vi "WriteTextFile.vi"(5 "overwrite? (F)":bool, 7 "InitialCali.":dbl[](array[numeric])=[-1.0, -1.0, -1.0], 8 "error in (no error)":errorcluster, 10 "Signal Segment":T1={"SampleRate"=-1.0, "TrigDelay"=0.0, "SpecLength"=0.0, "DAQ_Range"=0.0, "Average#"=0, "Position"=[], "Spectrum"=[], "Calibr."=[], "Pressure"=-1.0, "Desp_LaserEnergy"=-1.0, "PI_LaserEnergy"=-1.0, "Voltages Table"=[], "ProcMode"=enum."None", "Threshold"=-1.0, "Comment"="", "TickCount"=0.0, "Time Stamp"=timestamp(0 s since 1904-01-01)} {"TickCount" format="%#.2f"}, 11 "Filename":path) -> (0 "error out":errorcluster)   [LabVIEW 2013]
uses:
  Signal_Segment.ctl
  ControlDef/ProcessingMode.ctl
  <vilib>/Utility/error.llb/DialogType.ctl
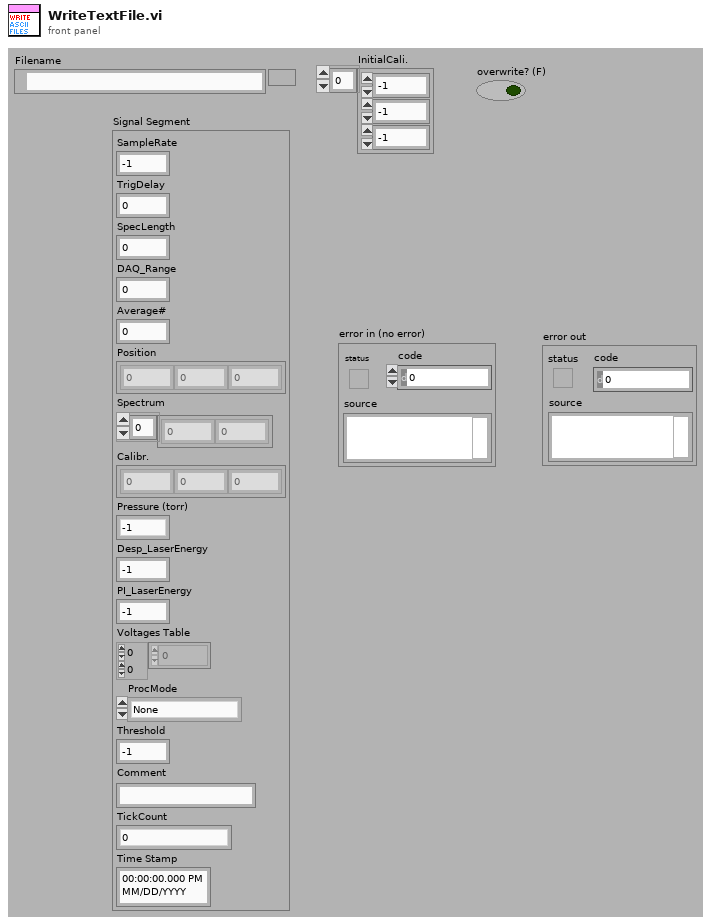
[diagram p1: front panel]
types:
  T1 = typedef "Signal_Segment.ctl" = cluster{"SampleRate":dbl, "TrigDelay":dbl, "SpecLength":dbl, "DAQ_Range":dbl, "Average#":i32, "Position":dbl[], "Spectrum":sgl[], "Calibr.":dbl[], "Pressure":dbl, "Desp_LaserEnergy":dbl, "PI_LaserEnergy":dbl, "Voltages Table":sgl[][], "ProcMode":T2, "Threshold":dbl, "Comment":string, "TickCount":dbl, "Time Stamp":timestamp}
  T2 = typedef "ProcessingMode.ctl" = enum16{"None", "Drop by Threshold", "TDC Simulate", "SetFilter"}
  T3 = enum16{"open", "replace", "create", "open or create", "replace or create", "replace or create with confirmation"}
  T4 = typedef "DialogType.ctl" = u16
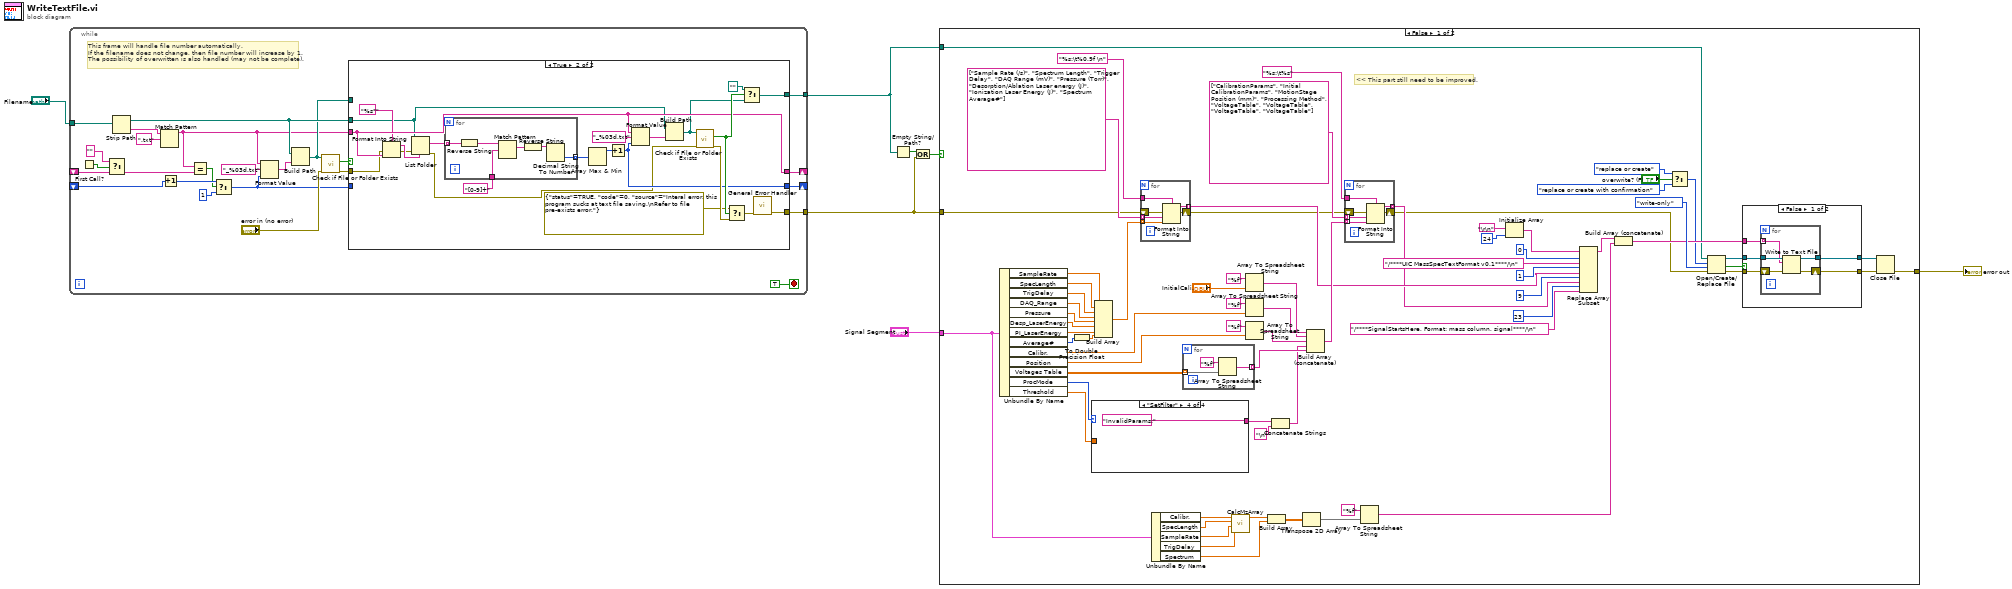
[diagram p0: block diagram]
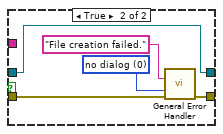
[diagram p3: hidden frame]
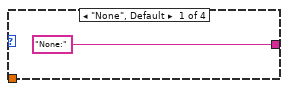
[diagram p4: hidden frame]
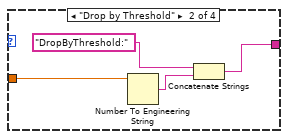
[diagram p5: hidden frame]
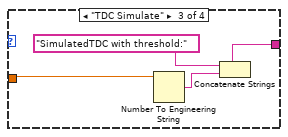
[diagram p6: hidden frame]
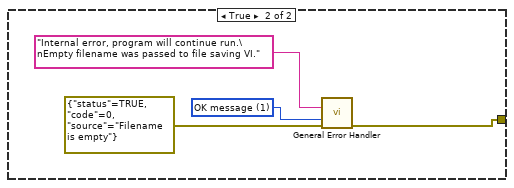
[diagram p7: hidden frame]
diagram:
  n1 = while {
    tunnel: "Filename" -> [w30]
    shift-right: [w23] -> _
    shift-left: _ -> [w10]
    shift-right: [w13] -> _
    shift-left: _ -> [w28]
    tunnel: [w21] -> w3
    tunnel: [w20] -> w1
    stop <- TRUE stop-if-true
    # "This frame will handle file number automatically.\nIf the filename does not change, then file number will increase by 1.\nThe possibility of overwritten is also handled (may not be complete)."
    n2 = First Call?() -> (First Call?: T/F=w9:bool)
    n3 = Select(t="", s=w9, f=w10) -> (s? t:f=w11:string)
    n4 = Strip Path(path=w30) -> (stripped path=w22:path, name=w32:string)
    n5 = Match Pattern(string=w32, regular expression=".txt") -> (before substring=w15:string)  [unwired: 1 in, 3 out]
    n6 = Increment(x=w28) -> (x+1=w27:i32)
    n7 = Equal?(x=w15, y=w11) -> (x = y?=w26:bool)
    n8 = Select(t=w27, s=w26, f=1) -> (s? t:f=w12:i32)
    n9 = Format Value(string ("")=w15, format string="_%03d.txt", value (0)=w12) -> (output string=w14:string)
    n10 = Build Path(base path=w22, name or relative path=w14) -> (appended path=w17:path)
    n11 = call <vilib>:"Check if File or Folder Exists.vi"("error in (no error)"="error in (no error)", "path"=w17) -> ("error out"=w19:errorcluster, "file or folder exists?"=w24:bool)  [unwired: 7 in, 1 out]
    n12 = case shown="True" w24 {
      tunnel: w22 -> [_ w37]
      tunnel: w15 -> [w36 w45]
      tunnel: [w36 w45] -> w23
      tunnel: w17 -> [w35 _]
      tunnel: [w35 w56] -> w21
      tunnel: [w34 w54] -> w20
      tunnel: w19 -> [w34 w42]
      tunnel: [w33 w46] -> w13
      tunnel: w12 -> [w33 _]
      frame False {
      }
      frame True {
        n13 = Format Into String(format string="%s*" ("initial string"), error in=w42, w45) -> (resulting string=w44:string, error out=w43:errorcluster)  [unwired: 1 in]
        n14 = List Folder(path=w37, pattern=w44, error in=w43) -> (filenames=w58:string[], error out=w41:errorcluster)  [unwired: 1 in, 2 out]
        n15 = for {
          tunnel: w58 -> [w64] mode=indexing
          tunnel: [w60] -> w57 mode=indexing
          tunnel: "[0-9]+" -> [w59]
          n16 = Reverse String(1:w64) -> (0:w63:string)
          n17 = Match Pattern(string=w63, regular expression=w59) -> (match substring=w62:string)  [unwired: 1 in, 3 out]
          n18 = Reverse String(1:w62) -> (0:w61:string)
          n19 = Decimal String To Number(string=w61) -> (number=w60:i32)  [unwired: 2 in, 1 out]
        }
        n20 = Array Max & Min(array=w57) -> (max value=w48:i32)  [unwired: 3 out]
        n21 = Increment(x=w48) -> (x+1=w46:i32)
        n22 = Format Value(string ("")=w45, format string="_%03d.txt", value (0)=w46) -> (output string=w47:string)
        n23 = Build Path(base path=w37, name or relative path=w47) -> (appended path=w38:path)
        n24 = call <vilib>:"Check if File or Folder Exists.vi"("error in (no error)"=w41, "path"=w38) -> ("error out"=w52:errorcluster, "file or folder exists?"=w51:bool)  [unwired: 7 in, 1 out]
        n25 = Select(t=errorcluster {"status"=TRUE, "code"=0, "source"="Interal error, this program sucks at text file saving.\nRefer to file pre-exists error."}, s=w51, f=w52) -> (s? t:f=w53:errorcluster)
        n26 = Select(t=path "", s=w51, f=w38) -> (s? t:f=w56:path)
        n27 = call <vilib>:"General Error Handler.vi"("error in (no error)"=w53) -> ("error out"=w54:errorcluster)  [unwired: 10 in, 4 out]
      }
    }
  }
  n28 = Empty String/Path?(string/path=w3) -> (empty?=w7:bool)
  n29 = Or(x=w7, y=w1) -> (x .or. y?=w2:bool)
  n30 = case shown="False" w2 {
    tunnel: "Signal Segment" -> [w82 _]
    tunnel: [w73 w175] -> w5
    tunnel: w1 -> [w83 _]
    tunnel: w3 -> [w81 _]
    frame False {
      # "<< This part still need to be improved."
      n31 = Unbundle By Name(w82) -> ("SampleRate"=w133:dbl, "SpecLength"=w132:dbl, "TrigDelay"=w131:dbl, "DAQ_Range"=w130:dbl, "Pressure"=w129:dbl, "Desp_LaserEnergy"=w128:dbl, "PI_LaserEnergy"=w127:dbl, "Average#"=w126:i32, "Calibr."=w120:dbl[], "Position"=w118:dbl[], "Voltages Table"=w89:sgl[][], "ProcMode"=w117:T2, "Threshold"=w116:dbl)
      n32 = To Double Precision Float(number=w126) -> (double precision float=w68:dbl)
      n33 = case shown="\"SetFilter\"" w117 {
        tunnel: ["None:" w156 w160 "InvalidParams:"] -> w79
        tunnel: w116 -> [_ w154 w158 _]
        frame "None", Default {
        }
        frame "Drop by Threshold" {
          n34 = Number To Engineering String(4:w154) -> (0:w157:string)  [unwired: 3 in]
          n35 = Concatenate Strings("DropByThreshold:", w157) -> (w156:string)
        }
        frame "TDC Simulate" {
          n36 = Number To Engineering String(4:w158) -> (0:w159:string)  [unwired: 3 in]
          n37 = Concatenate Strings("SimulatedTDC with threshold:", w159) -> (w160:string)
        }
        frame "SetFilter" {
        }
      }
      n38 = Build Array(w133, w132, w131, w130, w129, w128, w127, w68) -> (w125:dbl[])
      n39 = for {
        tunnel: string[] ["Sample Rate (/s)", "Spectrum Length", "Trigger Delay", "DAQ Range (mV)", "Pressure (Torr)", "Desorption/Ablation Laser energy (J)", "Ionization Laser Energy (J)", "Spectrum Average#"] -> [w174] mode=indexing
        tunnel: [w173] -> w92 mode=indexing
        tunnel: w125 -> [w172] mode=indexing
        tunnel: "%s:\t%0.9f \n" ("format string") -> [w171]
        shift-right: [w170] -> w84
        shift-left: w83 -> [w169]
        n40 = Format Into String(format string=w171, error in=w169, w174, w172) -> (resulting string=w173:string, error out=w170:errorcluster)  [unwired: 1 in]
      }
      n41 = Unbundle By Name(w82) -> ("Calibr."=w106:dbl[], "SpecLength"=w107:dbl, "SampleRate"=w108:dbl, "TrigDelay"=w109:dbl, "Spectrum"=w104:sgl[])
      n42 = for {
        tunnel: [w136] -> w80 mode=indexing
        tunnel: w89 -> [w135] mode=indexing
        n43 = Array To Spreadsheet String(array=w135, 3:"%f" ("format string")) -> (spreadsheet string=w136:string)  [unwired: 1 in]
      }
      n44 = call "CalcMzArray.vi"("TrigDelay"=w109, "Sample Rate"=w108, "Depth"=w107, "mzCali. (a/b/c)"=w106) -> ("mzArray"=w105:dbl[])  [unwired: 7 in]
      n45 = Array To Spreadsheet String(array="InitialCali.", 3:"%f" ("format string")) -> (spreadsheet string=w69:string)  [unwired: 1 in]
      n46 = Array To Spreadsheet String(array=w120, 3:"%f" ("format string")) -> (spreadsheet string=w114:string)  [unwired: 1 in]
      n47 = Array To Spreadsheet String(array=w118, 3:"%f" ("format string")) -> (spreadsheet string=w115:string)  [unwired: 1 in]
      n48 = Build Array(w105, w104) -> (w112:dbl[][])
      n49 = Concatenate Strings(w79, "\n" ("string")) -> (w78:string)
      n50 = Transpose 2D Array(2D array=w112) -> (transposed array=w110:dbl[][])
      n51 = Build Array (concatenate)(w114, w69, w115, w78, w80) -> (w113:string[])
      n52 = for {
        tunnel: string[] ["CalibrationParams", "Initial CalibrationParams", "MotionStage Position (mm)", "Processing Method", "VoltageTable", "VoltageTable", "VoltageTable", "VoltageTable"] -> [w168] mode=indexing
        tunnel: [w167] -> w90 mode=indexing
        tunnel: "%s:\t%s" ("format string") -> [w166]
        tunnel: w113 -> [w165] mode=indexing
        shift-right: [w164] -> w85
        shift-left: w84 -> [w163]
        n53 = Format Into String(format string=w166, error in=w163, w168, w165) -> (resulting string=w167:string, error out=w164:errorcluster)  [unwired: 1 in]
      }
      n54 = Array To Spreadsheet String(array=w110, 3:"%f" ("format string")) -> (spreadsheet string=w87:string)  [unwired: 1 in]
      n55 = Initialize Array("\r\n", 24 ("dimension size")) -> (w96:string[])
      n56 = Replace Array Subset(array=w96, new element #1="/****UIC MassSpecTextFormat v0.1****/\n" ("new element/subarray"), index #1=0 ("index"), new element #2=w92, index #2=1 ("index"), new element #3=w90, index #3=9 ("index"), new element #4="/****SignalStartsHere, Format: mass column, signal****/\n" ("new element/subarray"), index #4=23 ("index")) -> (w88:string[])
      n57 = Build Array (concatenate)(w88, w87) -> (w86:string[])
      n58 = Select(t=T3."replace or create", s="overwrite? (F)", f=T3."replace or create with confirmation" ("operation (0:open)")) -> (s? t:f=w67:T3)
      n59 = Open/Create/Replace File(file path (use dialog)=w81, error in=w85, operation (0:open)=w67, access (0:read/write)=enum16{"read/write", "read-only", "write-only"}."write-only") -> (refnum out=w99:refnum<file>, cancelled=w100:bool, error out=w103:errorcluster)  [unwired: 2 in]
      n60 = case shown="False" w100 {
        tunnel: w103 -> [w142 w149]
        tunnel: w99 -> [w141 w148]
        tunnel: w86 -> [w140 _]
        tunnel: [w139 w152] -> w74
        tunnel: [w138 w148] -> w72
        frame False {
          n61 = for {
            tunnel: w141 -> [w146]
            tunnel: w140 -> [w145] mode=indexing
            shift-right: [w144] -> w139
            shift-left: w142 -> [w147]
            tunnel: [w143] -> w138
            n62 = Write to Text File(file (use dialog)=w146, text=w145, error in=w147) -> (refnum out=w143:refnum<file>, error out=w144:errorcluster)  [unwired: 1 in, 1 out]
          }
        }
        frame True {
          w150 = T4 0 items=["no dialog", "OK message", "continue or stop message", "OK message + warnings", "continue/stop + warnings"] ("type of dialog (OK msg:1)")
          n63 = call <vilib>:"General Error Handler.vi"("[error source] (\" \")"="File creation failed." ("[error source] (\" \")"), "type of dialog (OK msg:1)"=w150, "error in (no error)"=w149) -> ("error out"=w152:errorcluster)  [unwired: 8 in, 4 out]
        }
      }
      n64 = Close File(refnum=w72, error in=w74) -> (error out=w73:errorcluster)  [unwired: 1 out]
    }
    frame True {
      w177 = T4 1 items=["no dialog", "OK message", "continue or stop message", "OK message + warnings", "continue/stop + warnings"] ("type of dialog (OK msg:1)")
      n65 = call <vilib>:"General Error Handler.vi"("[error source] (\" \")"="Internal error, program will continue run.\nEmpty filename was passed to file saving VI." ("[error source] (\" \")"), "type of dialog (OK msg:1)"=w177, "error in (no error)"=errorcluster {"status"=TRUE, "code"=0, "source"="Filename is empty"} ("error out")) -> ("error out"=w175:errorcluster)  [unwired: 8 in, 4 out]
    }
  }
  "error out" <- w5
